vi "op_num_v1.vi"() -> ()   [LabVIEW 2009]
panel:
  out "N: numar aleator":dbl format="%.3f"
  out "Afisor numeric":i32
  # "- se genereaza un numar aleator N\n- valoarea lui N este cuprinsa intre 0-1\n- se calculeaza produsul  N*1000 \n- se afiseaza rezultatul"
  # "Produsul N*1000 este:"
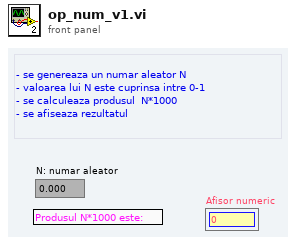
[diagram p1: front panel]
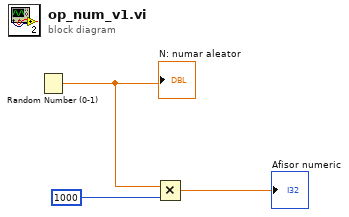
[diagram p0: block diagram]
diagram:
  n1 = Random Number (0-1)() -> (number: 0 to 1=w2:dbl)
  "N: numar aleator" <- w2
  n2 = Multiply(x=w2, y=1000) -> (x*y=→"Afisor numeric":dbl)
